vi "TDMS2TDMCreateChannel.vi"(8 "error in (no error)":errorcluster, 9 "Object type":string="tdm_channelgroup", 10 "Name":string, 11 "Data Object":refnum<k20>) -> (0 "error out":errorcluster, 2 "New Storage Refnum":refnum<k20>, 3 "dup storage refnum":refnum<k20>)   [LabVIEW 2017]
doc: "This VI creates a new channel or channel group as a child object of the Data Object input. It checks that a valid name is given and coerces the name if necessary to fit the TDM storage format."
uses:
  <vilib>/Utility/tdmsutil.llb/TDMS2TDMNameType.ctl
  <vilib>/Platform/storage/Storage.llb/__savePropString.vi
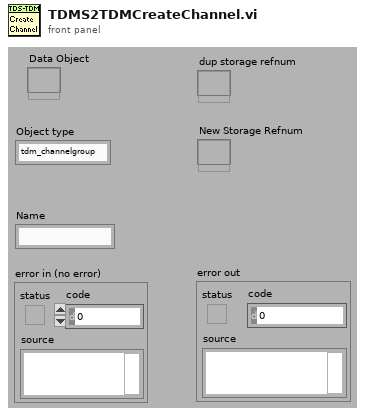
[diagram p1: front panel]
types:
  T1 = typedef "TDMS2TDMNameType.ctl" = enum16{"Channel", "Property"}
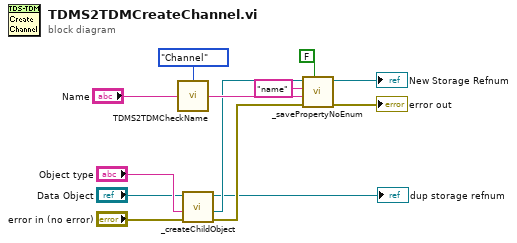
[diagram p0: block diagram]
diagram:
  n1 = call <vilib>:"TDMS2TDMCheckName.vi"("Name Type"=TDMS2TDMNameType."Channel", "Name"="Name") -> ("Name Out"=w10:string)  [unwired: 13 in]
  n2 = call <vilib>:"_createChildObject.vi"("error in (no error)"="error in (no error)", "Object type"="Object type", "storage refnum"="Data Object") -> ("error out"=w12:errorcluster, "new storage refnum"=w6:refnum<k20>, "dup storage refnum"=→"dup storage refnum":refnum<k20>)  [unwired: 2 in]
  n3 = call-poly <vilib>:"_savePropertyNoEnum.vi"("User-defined property"=FALSE, "error in (no error)"=w12, "Value"=w10, "Property name"="name" ("Object type"), "storage refnum"=w6) -> ("error out"=→"error out":errorcluster, "dup storage refnum"=→"New Storage Refnum":refnum<k20>)  [unwired: 5 in]
